vi "Init Sub VI GLD.vi"(0 "Weight":T6, 1 "Patient ID":string caption="Participant Name (FirstLast)", 2 "Group ID":T5, 3 "Hand in Test":T4 caption="Test Type", 4 "Trial":string caption="Participant Name (FirstLast)", 5 "String 3":string, 6 "Test Type":T7, 7 "Ramp's Height (N)":T1, 9 "Ramp's Width (s)":T3 caption="Test Type", 13 "Wrist Angle":enum16{"0", "30", "-30"}(ring), 19 "Sine Min/Max":T2=3000.0) -> (14 "Lab2Ardu":string, 16 "Foldername and filename string":string, 17 "Ramp's Width":dbl, 18 "Ramp's Height":dbl)   [LabVIEW 2019]
uses:
  weightTypedef.ctl
  groupID.ctl
  handInTest.ctl
  TESTtypedef UPDATED.ctl
  RampSlope.ctl
  SineMinMax.ctl
  RampHeight.ctl
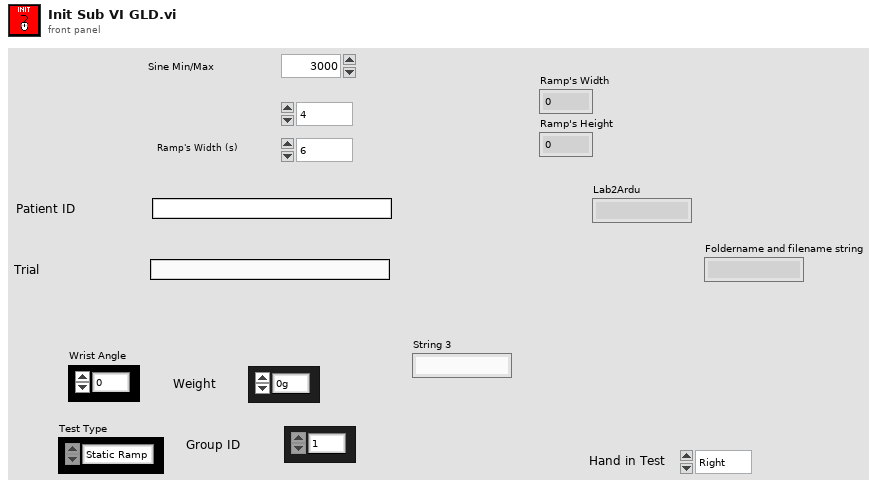
[diagram p1: front panel]
types:
  T1 = typedef "RampHeight.ctl" = enum16{"4", "5", "6"}
  T2 = typedef "SineMinMax.ctl" = dbl
  T3 = typedef "RampSlope.ctl" = enum16{"6", "5", "4"}
  T4 = typedef "handInTest.ctl" = enum16{"Right", "Left"}
  T5 = typedef "groupID.ctl" = enum16{"1", "2"}
  T6 = typedef "weightTypedef.ctl" = enum16{"0g", "300g", "600g", "900g"}
  T7 = typedef "TESTtypedef UPDATED.ctl" = enum16{"Static Ramp", "Static Sine", "Dynamic"}
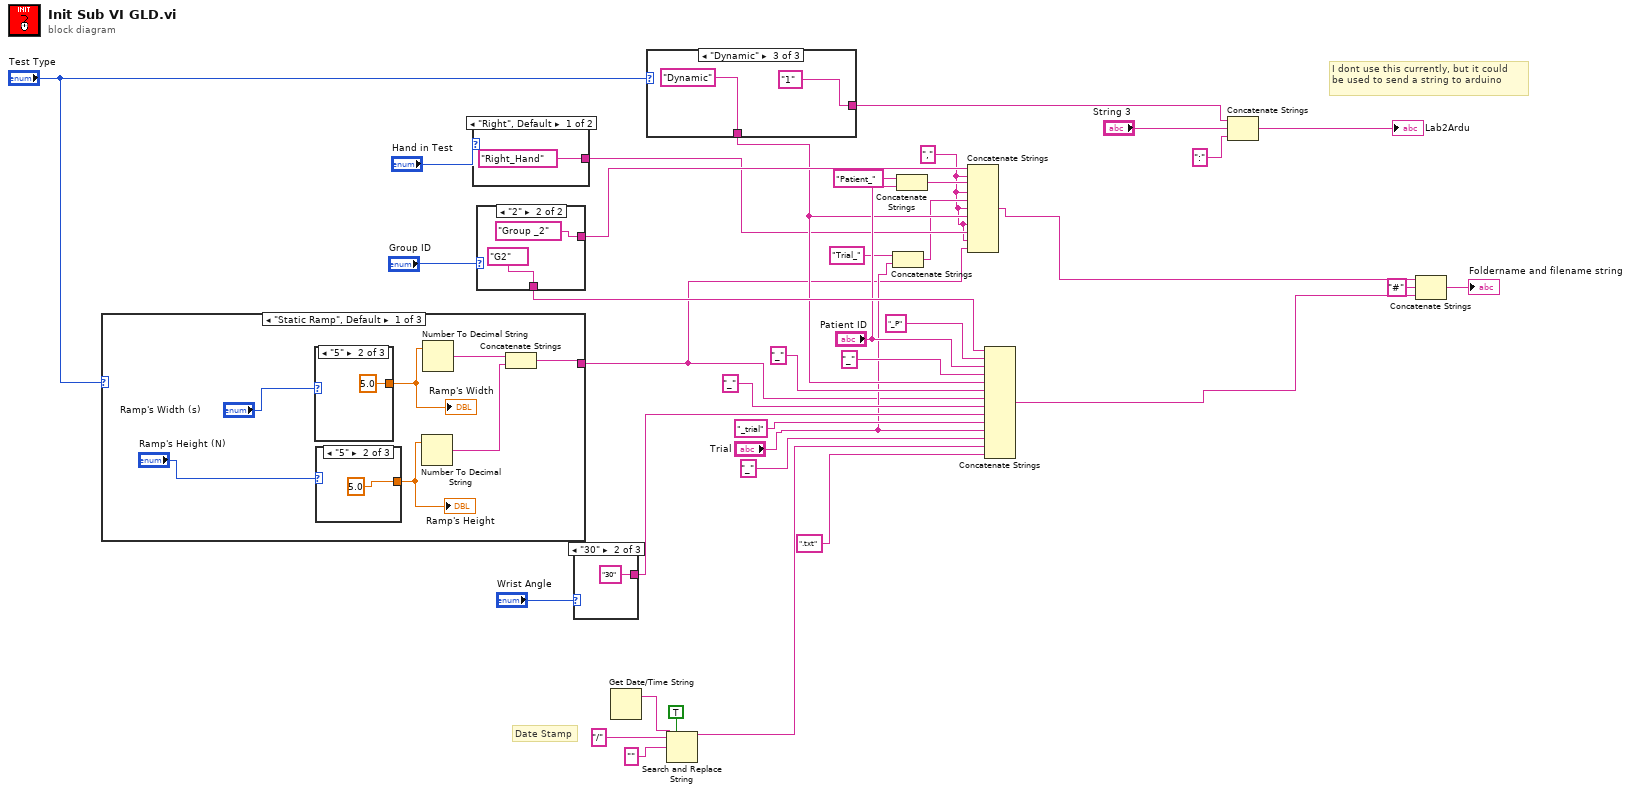
[diagram p0: block diagram]
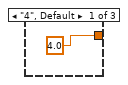
[diagram p2: hidden frame]
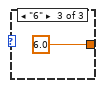
[diagram p3: hidden frame]
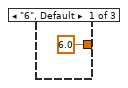
[diagram p4: hidden frame]
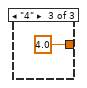
[diagram p5: hidden frame]
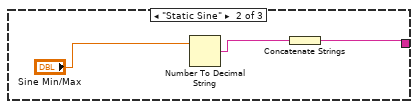
[diagram p6: hidden frame]
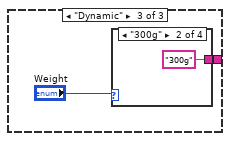
[diagram p7: hidden frame]
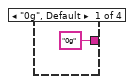
[diagram p8: hidden frame]
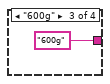
[diagram p9: hidden frame]
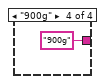
[diagram p10: hidden frame]
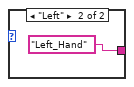
[diagram p11: hidden frame]
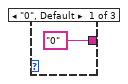
[diagram p12: hidden frame]
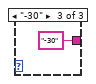
[diagram p13: hidden frame]
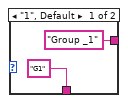
[diagram p14: hidden frame]
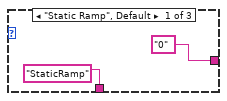
[diagram p15: hidden frame]
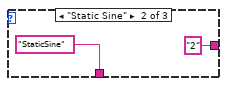
[diagram p16: hidden frame]
diagram:
  w7 = "," ("string")
  # "I dont use this currently, but it could \nbe used to send a string to arduino"
  # "Date Stamp"
  n1 = case shown="\"Static Ramp\", Default" "Test Type" {
    tunnel: [w44 w51 w54] -> w6
    frame "Static Ramp", Default {
      n2 = case shown="\"5\"" "Ramp's Width (s)" {
        tunnel: [6.0 5.0 4.0] -> w41
        frame "6", Default {
        }
        frame "5" {
        }
        frame "4" {
        }
      }
      "Ramp's Width" <- w41
      n3 = case shown="\"5\"" "Ramp's Height (N)" {
        tunnel: [4.0 5.0 6.0] -> w39
        frame "4", Default {
        }
        frame "5" {
        }
        frame "6" {
        }
      }
      "Ramp's Height" <- w39
      n4 = Number To Decimal String(number=w39) -> (decimal integer string=w38:string)  [unwired: 1 in]
      n5 = Number To Decimal String(number=w41) -> (decimal integer string=w43:string)  [unwired: 1 in]
      n6 = Concatenate Strings(w43, w38) -> (w44:string)
    }
    frame "Static Sine" {
      n7 = Number To Decimal String(number="Sine Min/Max") -> (decimal integer string=w52:string)  [unwired: 1 in]
      n8 = Concatenate Strings(w52) -> (w51:string)
    }
    frame "Dynamic" {
      n9 = case shown="\"300g\"" "Weight" {
        tunnel: ["0g" "300g" "600g" "900g"] -> w54
        frame "0g", Default {
        }
        frame "300g" {
        }
        frame "600g" {
        }
        frame "900g" {
        }
      }
    }
  }
  n10 = case shown="\"Right\", Default" "Hand in Test" {
    tunnel: ["Right_Hand" "Left_Hand"] -> w11
    frame "Right", Default {
    }
    frame "Left" {
    }
  }
  n11 = case shown="\"2\"" "Group ID" {
    tunnel: ["G1" "G2"] -> w28
    tunnel: ["Group _1" "Group _2"] -> w18
    frame "1", Default {
    }
    frame "2" {
    }
  }
  n12 = case shown="\"30\"" "Wrist Angle" {
    tunnel: ["0" "30" "-30"] -> w23
    frame "0", Default {
    }
    frame "30" {
    }
    frame "-30" {
    }
  }
  n13 = Get Date/Time String() -> (date string=w29:string)  [unwired: 3 in, 1 out]
  n14 = case shown="\"Dynamic\"" "Test Type" {
    tunnel: ["0" "2" "1"] -> w36
    tunnel: ["StaticRamp" "StaticSine" "Dynamic"] -> w13
    frame "Static Ramp", Default {
    }
    frame "Static Sine" {
    }
    frame "Dynamic" {
    }
  }
  n15 = Search and Replace String(replace all?=TRUE ("replace all? (F)"), input string=w29, search string="/", replace string="" ("replace string (\"\")")) -> (result string=w20:string)  [unwired: 4 in, 3 out]
  n16 = Concatenate Strings("Trial_" ("string"), "Trial") -> (w8:string)
  n17 = Concatenate Strings("Patient_" ("string"), "Patient ID") -> (w15:string)
  n18 = Concatenate Strings(w18, w7, w15, w7, w8, w7, w13, w7, w11, w7, w6) -> (w4:string)
  n19 = Concatenate Strings(w28, "_P" ("string"), "Patient ID", "_" ("string"), w13, "_" ("string"), w6, "_" ("string"), w23, "_trial" ("string"), "Trial", "_" ("string"), w20, ".txt" ("string")) -> (w2:string)
  n20 = Concatenate Strings(w36, "String 3", ":" ("string")) -> (→"Lab2Ardu":string)
  n21 = Concatenate Strings(w4, "#" ("string"), w2) -> (→"Foldername and filename string":string)
